vi "LV to ITX Retrieve_SE mode.vi"(0 "File or Folder Path":path=path "G:/My Drive/ansom/Data/MNK/SA03018F.20180502/4 - sweep B, Vsg IV superlattice", 5 "offset":i32, 7 "length":i32=1, 9 "index":T3={"A"=7, "B"=5, "C"=3, "D"=5, "E"=3, "N1"=2, "N2"=2, "N3"=3, "N4"=4, "A 1"=4, "A 2"=6, "C 1"=3, "C 2"=1, "E 2"=4}, 11 "stop":bool, 12 "File Type":T1) -> (1 "Spherical coordinates":dbl[][](array[numeric]), 2 "long":cluster{i32[], dbl[]}(graph), 3 "G vs T":cluster{dbl[], dbl[]}(graph), 4 "A vs B":cluster{dbl[], dbl[]}[](graph), 6 "C vs D":cluster{dbl[], dbl[]}[](graph), 8 "E( = A)":dbl[][](graph), 10 "N":cluster{"N1":dbl, "N2":dbl, "N3":dbl, "N4":dbl}={"N1"=17.9999, "N2"=17.9999, "N3"=0.00140599360448446, "N4"=0.001168874519263091} {"N4" format="%#_6p"; "N3" format="%#_6p"; "N2" format="%#_6p"; "N1" format="%#_6p"}, 13 "Index, Wavenames":string[][](table)=[["0", "'time.SA03018F.20180502.000000'\n"], ["1", "'temp.SA03018F.20180502.000000'\n"], ["2", "'B.SA03018F.20180502.000000'\n"], ["3", "'Vsource.SA03018F.20180502.000000'\n"], ["4", "'Lockin0.SA03018F.20180502.000000'\n"], ["5", "'Lockin1.SA03018F.20180502.000000'\n"], ["6", "'Lockin2.SA03018F.20180502.000000'\n"], ["7", "'Lockin3.SA03018F.20180502.000000'\n"], ["8", "'Lockin4.SA03018F.20180502.000000'\n"], ["9", "'Lockin5.SA03018F.20180502.000000'\n"], ["10", "'B_rate.SA03018F.20180502.000000'\n"], ["11", "'DC0.SA03018F.20180502.000000'\n"], ["12", "'DC1.SA03018F.20180502.000000'\n"], ["13", "'DC2.SA03018F.20180502.000000'\n"], ["14", "'DC3.SA03018F.20180502.000000'\n"], ["15", "'DC4.SA03018F.20180502.000000'\n"], ["16", "'DC5.SA03018F.20180502.000000'\n"], ["17", "'DC6.SA03018F.20180502.000000'\n"], ["18", "'DC7.SA03018F.20180502.000000'\n"], ["", ""]], 14 "Comments":string="IGOR\nX// Date: 5/3/2018 12:09 PM\nX// B=18T to -18T 0.5T steps\nX// T=30mK\nX// sweep Vsg -10mV --> 60mV, 0.25mV step\nX// Vsg=1.1V\nX// \nX// lockin settings:\nX// time constant =100ms\nX// order=2\nX// Fs=2000\nX// #s=5000\nX// \nX// superlattice\nX// \nX// lockin:\nX// 0: 4, voltage V+\nX// 1: 5, current 8mV AC 270uV DC, 0.4 Hz\nX// 2: 7, voltage V-\nX// 3: 3, current, drain\nX// 4: 2,\nX// 5: 1, \nX// appliedField= 18.000000\nX// appliedVsg= -0.010000\nX// B= 17.999900\n\n\n\n\n\n\n\n\n\n\n\n\n\n\n\n\n\n\n\n\n\n\n\n\n\n\n\n\n\n\n\n\n\n\n\n\n\n\n\n\nX \nX Display/R 'time.SA03018F.20180502.000000'\nX AppendToGraph 'temp.SA03018F.20180502.000000'\nX AppendToGraph 'B.SA03018F.20180502.000000'\nX AppendToGraph 'Vsource.SA03018F.20180502.000000'\nX AppendToGraph 'Lockin0.SA03018F.20180502.000000'\nX AppendToGraph 'Lockin1.SA03018F.20180502.000000'\nX AppendToGraph 'Lockin2.SA03018F.20180502.000000'\nX AppendToGraph 'Lockin3.SA03018F.20180502.000000'\nX AppendToGraph 'Lockin4.SA03018F.20180502.000000'\nX AppendToGraph 'Lockin5.SA03018F.20180502.000000'\nX AppendToGraph 'B_rate.SA03018F.20180502.000000'\nX AppendToGraph 'DC0.SA03018F.20180502.000000'\nX AppendToGraph 'DC1.SA03018F.20180502.000000'\nX AppendToGraph 'DC2.SA03018F.20180502.000000'\nX AppendToGraph 'DC3.SA03018F.20180502.000000'\nX AppendToGraph 'DC4.SA03018F.20180502.000000'\nX AppendToGraph 'DC5.SA03018F.20180502.000000'\nX AppendToGraph 'DC6.SA03018F.20180502.000000'\nX AppendToGraph 'DC7.SA03018F.20180502.000000'\nX Label bottom \"x label\"\nX Label left \"y label\"\nX ModifyGraph rgb('time.SA03018F.20180502.000000')=(65280,0,0)\nX ModifyGraph rgb('temp.SA03018F.20180502.000000')=(65280,18432,0)\nX ModifyGraph rgb('B.SA03018F.20180502.000000')=(65280,36864,0)\nX ModifyGraph rgb('Vsource.SA03018F.20180502.000000')=(65280,55296,0)\nX ModifyGraph rgb('Lockin0.SA03018F.20180502.000000')=(57344,65280,0)\nX ModifyGraph rgb('Lockin1.SA03018F.20180502.000000')=(37376,65280,0)\nX ModifyGraph rgb('Lockin2.SA03018F.20180502.000000')=(18944,65280,0)\nX ModifyGraph rgb('Lockin3.SA03018F.20180502.000000')=(512,65280,0)\nX ModifyGraph rgb('Lockin4.SA03018F.20180502.000000')=(0,65280,17920)\nX ModifyGraph rgb('Lockin5.SA03018F.20180502.000000')=(0,65280,36352)\nX ModifyGraph rgb('B_rate.SA03018F.20180502.000000')=(0,65280,54784)\nX ModifyGraph rgb('DC0.SA03018F.20180502.000000')=(0,57856,65280)\nX ModifyGraph rgb('DC1.SA03018F.20180502.000000')=(0,39424,65280)\nX ModifyGraph rgb('DC2.SA03018F.20180502.000000')=(0,20992,65280)\nX ModifyGraph rgb('DC3.SA03018F.20180502.000000')=(0,2560,65280)\nX ModifyGraph rgb('DC4.SA03018F.20180502.000000')=(17408,0,65280)\nX ModifyGraph rgb('DC5.SA03018F.20180502.000000')=(35840,0,65280)\nX ModifyGraph rgb('DC6.SA03018F.20180502.000000')=(54272,0,65280)\nX ModifyGraph rgb('DC7.SA03018F.20180502.000000')=(65280,0,58368)\nX Legend/C/N=text0/J \"\\\\s('time.SA03018F.20180502.000000') time\\r\\\\s('temp.SA03018F.20180502.000000') temp\\r\\\\s('B.SA03018F.20180502.000000') B\\r\\\\s('Vsource.SA03018F.20180502.000000') Vsource\\r\\\\s('Lockin0.SA03018F.20180502.000000') Lockin0\\r\\\\s('Lockin1.SA03018F.20180502.000000') Lockin1\\r\\\\s('Lockin2.SA03018F.20180502.000000') Lockin2\\r\\\\s('Lockin3.SA03018F.20180502.000000') Lockin3\\r\\\\s('Lockin4.SA03018F.20180502.000000') Lockin4\\r\\\\s('Lockin5.SA03018F.20180502.000000') Lockin5\\r\\\\s('B_rate.SA03018F.20180502.000000') B_rate\\r\\\\s('DC0.SA03018F.20180502.000000') DC0\\r\\\\s('DC1.SA03018F.20180502.000000') DC1\\r\\\\s('DC2.SA03018F.20180502.000000') DC2\\r\\\\s('DC3.SA03018F.20180502.000000') DC3\\r\\\\s('DC4.SA03018F.20180502.000000') DC4\\r\\\\s('DC5.SA03018F.20180502.000000') DC5\\r\\\\s('DC6.SA03018F.20180502.000000') DC6\\r\\\\s('DC7.SA03018F.20180502.000000') DC7\"\nX ModifyGraph mirror(bottom)=1\nX ModifyGraph width=216\nX ModifyGraph height={Aspect,0.6}\nX ModifyGraph Log(bottom)=0\nX ModifyGraph Log(left)=0\nX \n", 15 "E index vs Field":cluster{i32[], dbl[]}(graph))   [LabVIEW 2016, in "Retrieve and Visualize.lvclass"]
uses:
  Retrieve and Visualize.lvclass
  <vilib>/Utility/miscctls.llb/LVOffsetAndMultiplierTypeDef.ctl
  <userlib>/LevyLab/LV to ITX/Data/Typedefs/File Type--enum.ctl
  <vilib>/Analysis/3filter.llb/Savitzky-Golay Filter (DBL).vi
  <userlib>/LevyLab/XY Utilities/subVIs/Subset (single).vi
  <userlib>/LevyLab/XY Utilities/subVIs/Derivative (single).vi
  <userlib>/LevyLab/XY Utilities/subVIs/Decimate (single).vi
  <userlib>/LevyLab/Graph Utilities/graph_utilities.lvclass
  <vilib>/Analysis/NI_AALPro.lvlib
  <vilib>/Analysis/NI_AALBase.lvlib
  <userlib>/LevyLab/LV to ITX/Data/Data.lvclass
  <userlib>/LevyLab/XY Utilities/xy_utilities.lvlib
panel:
  out "Date":dbl format="%<%I:%M:%S %p\n%x>T"
  in  "Type":enum16{"dy/dx vs x", "dx/dy vs y"}(ring)
  in  "VRM mode":bool
  in  "Ring":u16(ring) items=["default", "DIFF"]
  in  "decimating factor":i32=1
  in  "decimate files":i32=1
  in  "side points":i32=6
  in  "fit points":dbl=10.0
  in  "Portion of data":cluster{dbl, dbl}(slide)={0.75, 0.25} scale=0.0..1.0
  in  "length 2":i32=2500
  in  "index 2":i32=1072
  out "Ns":T2(array[cluster])
  in  "SE?":bool=TRUE
  in  "D  is time?":bool
  in  "B is time?":bool
  in  "Ez name":string="Conductance (S)"
  in  "Ey name":string="BY (T)"
  in  "Ex name":string="Vsg (mV)"
  in  "C y name":string="voltage"
  in  "D x name":string="Vsg"
  in  "A y name":string="current"
  in  "B x name":string="Vsg"
  in  "recolor traces?":bool
  in  "Ex":T4={"Offset"=0.0, "Multiplier"=1.0}
  in  "Ey":T4={"Offset"=0.0, "Multiplier"=1.0}
  out "Path":path=path "G:/My Drive/ansom/Data/MNK/SA03018F.20180502/4 - sweep B, Vsg IV superlattice/SA03018F.20180502.000000.itx"
  out "counter":i32
  # "A1-A2\nC1-C2\nE-E2"
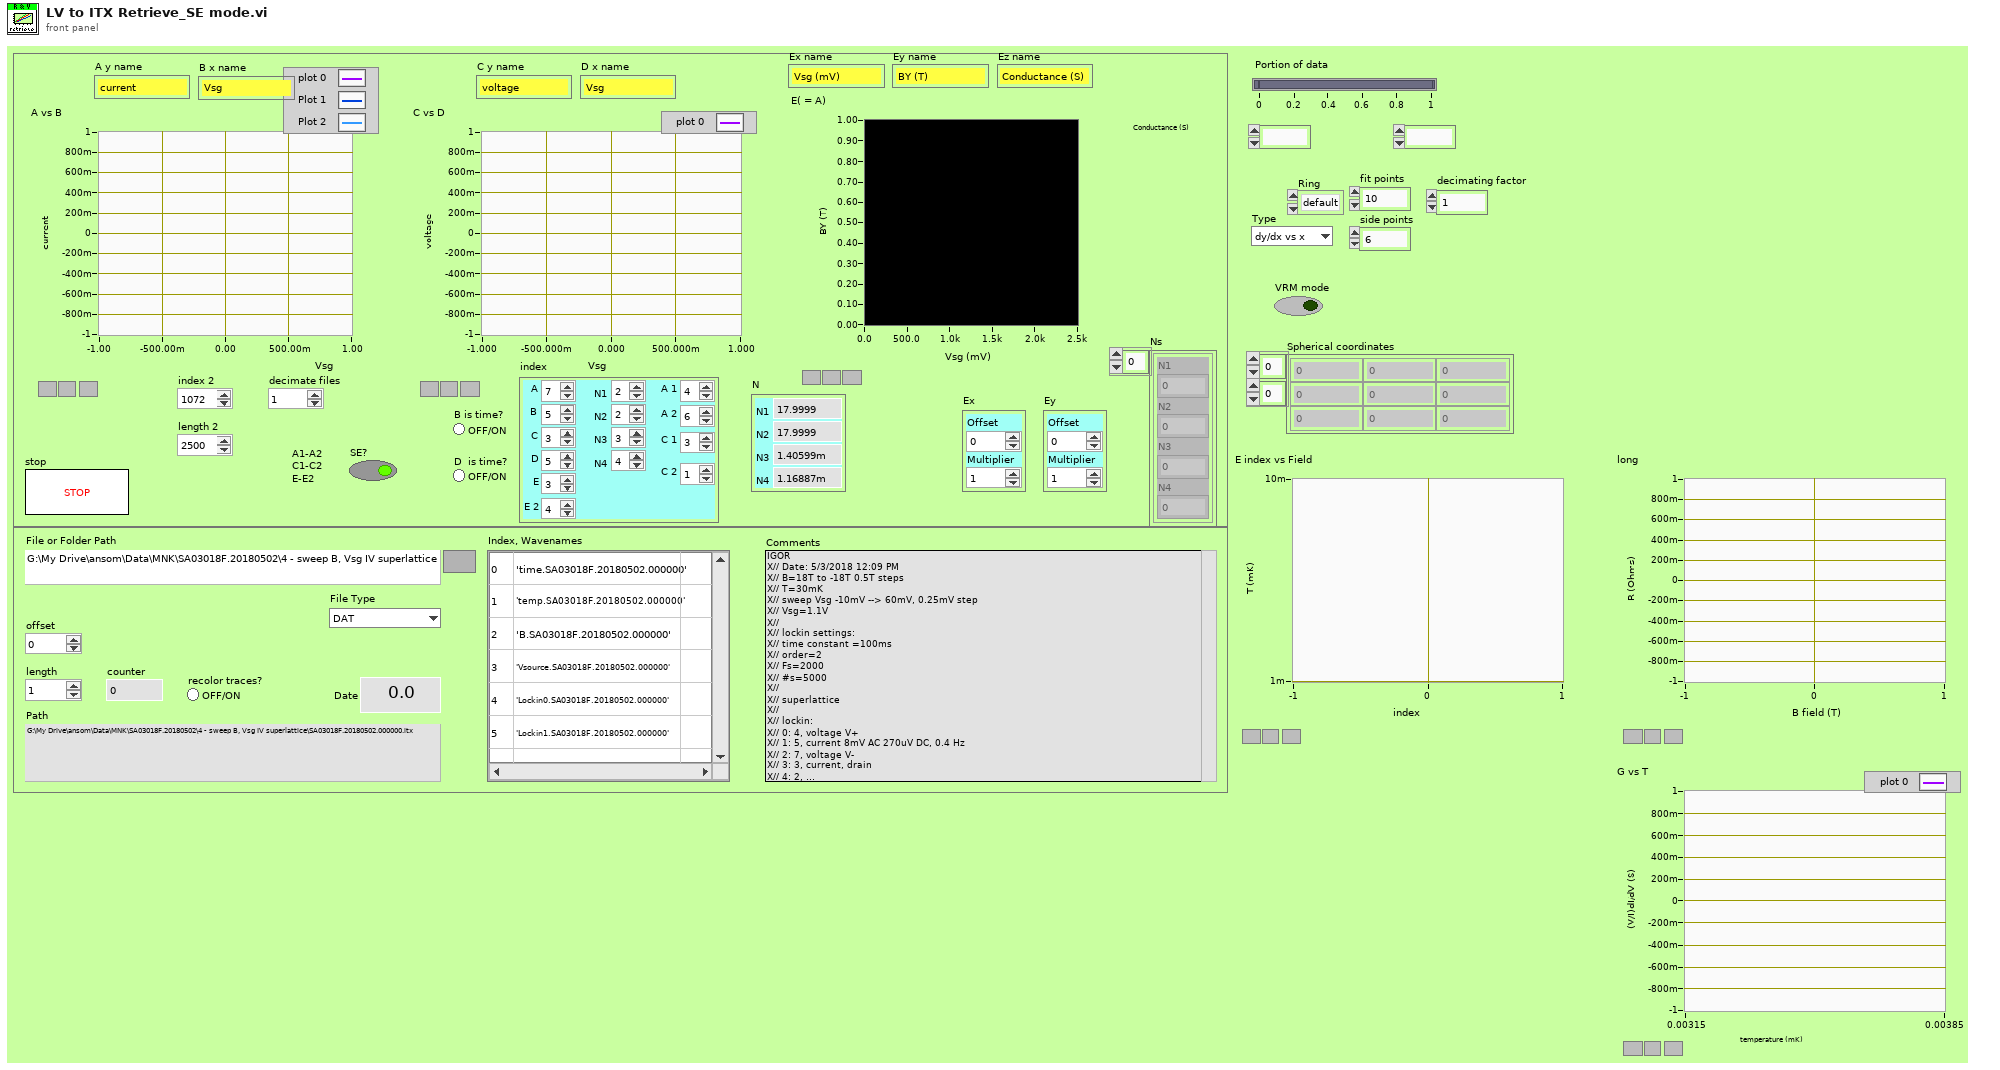
[diagram p1: front panel]
types:
  T1 = typedef "Data.lvclass/File Type--enum.ctl" = enum16{"DAT", "ITX", "TDMS", "VI"}
  T2 = cluster{"N1":dbl, "N2":dbl, "N3":dbl, "N4":dbl}[]
  T3 = cluster{"A":i32, "B":i32, "C":i32, "D":i32, "E":i32, "N1":i32, "N2":i32, "N3":i32, "N4":i32, "A 1":i32, "A 2":i32, "C 1":i32, "C 2":i32, "E 2":i32}
  T4 = typedef "LVOffsetAndMultiplierTypeDef.ctl" = cluster{"Offset":dbl, "Multiplier":dbl}
  T5 = typedef "Data.lvclass/Dictionary--cluster.ctl" = cluster{"key":string, "value":variant}
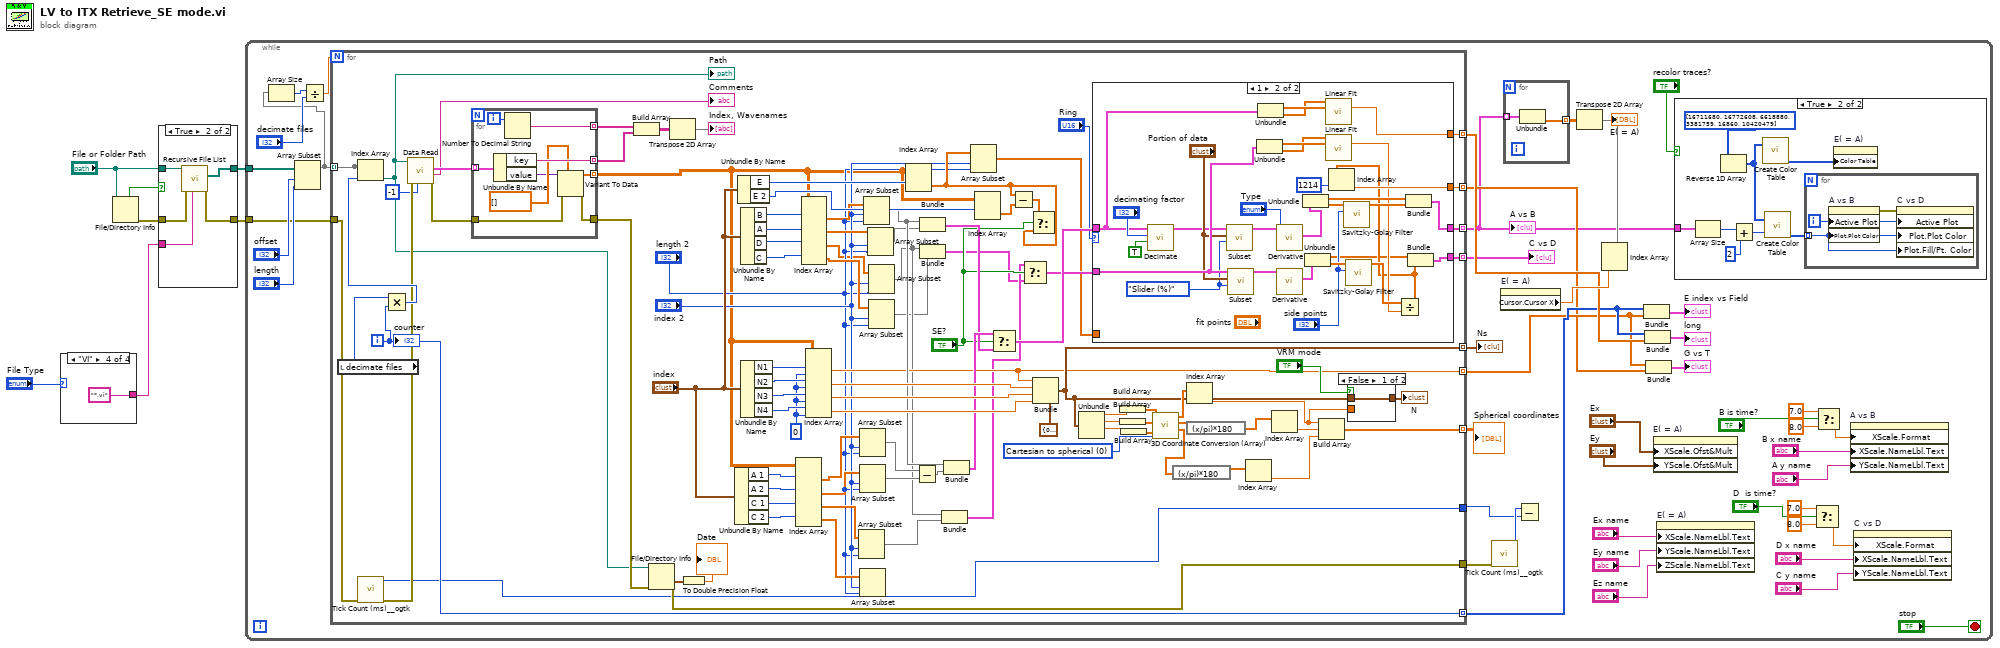
[diagram p0: block diagram]
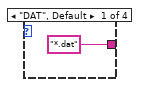
[diagram p2: hidden frame]
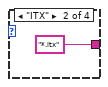
[diagram p3: hidden frame]
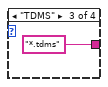
[diagram p4: hidden frame]
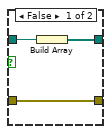
[diagram p5: hidden frame]
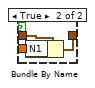
[diagram p7: hidden frame]
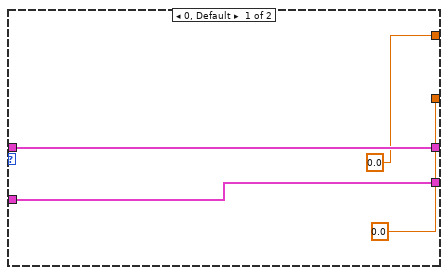
[diagram p8: hidden frame]
diagram:
  n1 = case shown="\"VI\"" "File Type" {
    tunnel: ["*.dat" ("pattern") "*.itx" ("pattern") "*.tdms" ("pattern") "*.vi" ("pattern")] -> w1
    frame "DAT", Default {
    }
    frame "ITX" {
    }
    frame "TDMS" {
    }
    frame "VI" {
    }
  }
  n2 = File/Directory Info(path="File or Folder Path") -> (directory=w5:bool, error out=w3:errorcluster)  [unwired: 1 in, 5 out]
  n3 = case shown="True" w5 {
    tunnel: [w14 w15] -> w6
    tunnel: "File or Folder Path" -> [w13 w19]
    tunnel: [w12 w18] -> w4
    tunnel: w3 -> [w12 w17]
    tunnel: w1 -> [_ w16]
    frame False {
      n4 = Build Array(w13) -> (w14:path[])
    }
    frame True {
      n5 = call <vilib>:"Recursive File List.vi"("pattern"=w16, "error in (no error)"=w17, "Folder Path"=w19) -> ("error out"=w18:errorcluster, "All Files in Dir"=w15:path[])  [unwired: 4 in, 3 out]
    }
  }
  n6 = while {
    tunnel: w6 -> [w41]
    tunnel: w4 -> [w24]
    stop <- "stop" stop-if-true
    n7 = Array Subset(array=w41, index="offset", length="length") -> (w37:path[])
    n8 = Array Size(array=w37) -> (size(s)=w40:i32)
    n9 = Divide(x=w40, y="decimate files") -> (x/y=w38:dbl)
    n10 = for {
      N: w38 -> [_]
      tunnel: w37 -> [w171]
      tunnel: [w171] -> _ mode=indexing
      tunnel: [w117] -> w25 mode=indexing
      tunnel: [w116] -> w26 mode=indexing
      tunnel: [w106] -> w44 mode=indexing
      tunnel: [w115] -> w42 mode=indexing
      tunnel: [w110] -> w34 mode=indexing
      tunnel: [w109] -> w27 mode=indexing
      tunnel: [w103] -> w31 mode=indexing
      tunnel: [w102] -> w30 mode=indexing
      tunnel: w24 -> [w84]
      tunnel: [w82] -> w22
      tunnel: [w81] -> w20
      i -> [w103]
      w132 = u16 0 items=["Cartesian to spherical", "spherical to Cartesian", "Cartesian to cylindrical", "cylindrical to Cartesian", "spherical to cylindrical", "cylindrical to spherical"] ("conversion type")
      w154 = 0 ("disabled index (col)")
      n11 = local read "decimate files"() -> (w113:i32)
      n12 = call <userlib>:"Tick Count (ms)__ogtk.vi"("error in (no error)"=w84) -> ("error out"=w83:errorcluster, "millisecond timer value"=w81:u32)  [unwired: 9 in]
      n13 = Multiply(x=w113, y=w103) -> (x*y=w114:i32)
      n14 = Index Array(array=w171, index=w114) -> (element=w79:path)
      "Path" <- w79
      n15 = call <userlib>:"Data Read.vi"("Append Index"=-1, "error in (no error)"=w83, "path"=w79) -> ("error out"=w89:errorcluster, "Notes"=→"Comments":string, "Data (Dictionary)"=w91:T5[])  [unwired: 5 in, 1 out]
      n16 = for {
        tunnel: [w179] -> w87 mode=indexing
        tunnel: w91 -> [w178] mode=indexing
        tunnel: [w177] -> w86 mode=indexing
        tunnel: [w175] -> w88 mode=indexing
        tunnel: w89 -> [w173]
        tunnel: [w172] -> w85
        i -> [w180]
        n17 = Unbundle By Name(w178) -> ("key"=w177:string, "value"=w174:variant)
        n18 = Number To Decimal String(number=w180) -> (decimal integer string=w179:string)  [unwired: 1 in]
        n19 = Variant To Data(error in=w173, type=dbl[] [], Variant=w174) -> (data=w175:dbl[], error out=w172:errorcluster)
      }
      n20 = Build Array(w87, w86) -> (w169:string[][])
      n21 = File/Directory Info(path=w79, error in=w85) -> (last mod=w78:timestamp, error out=w82:errorcluster)  [unwired: 5 out]
      n22 = Transpose 2D Array(2D array=w169) -> (transposed array=→"Index, Wavenames":string[][])
      n23 = To Double Precision Float(number=w78) -> (double precision float=→"Date":dbl)
      n24 = Unbundle By Name("index") -> ("A 1"=w153:i32, "A 2"=w152:i32, "C 1"=w151:i32, "C 2"=w150:i32)
      n25 = Unbundle By Name("index") -> ("E"=w162:i32, "E 2"=w145:i32)
      n26 = Unbundle By Name("index") -> ("B"=w161:i32, "A"=w160:i32, "D"=w159:i32, "C"=w158:i32)
      n27 = Unbundle By Name("index") -> ("N1"=w163:i32, "N2"=w164:i32, "N3"=w165:i32, "N4"=w166:i32)
      n28 = Index Array(array=w88, index (row) #1=w153, index (row) #2=w152, index (row) #3=w151, index (row) #4=w150) -> (element #1=w137:dbl[], element #2=w135:dbl[], element #3=w134:dbl[], element #4=w133:dbl[])  [unwired: 4 in]
      n29 = Index Array(array=w88, index (row) #1=w161, index (row) #2=w160, index (row) #3=w159, index (row) #4=w158) -> (element #1=w142:dbl[], element #2=w140:dbl[], element #3=w93:dbl[], element #4=w138:dbl[])  [unwired: 4 in]
      n30 = Index Array(array=w88, index (row) #1=w163, index (col) #1=w154, index (row) #2=w164, index (col) #2=w154, index (row) #3=w165, index (col) #3=w154, index (row) #4=w166, index (col) #4=w154) -> (element #1=w102:dbl, element #2=w156:dbl, element #3=w157:dbl, element #4=w168:dbl)
      n31 = Array Subset(array=w134, index="index 2", length="length 2") -> (w101:dbl[])
      n32 = Array Subset(array=w137, index="index 2", length="length 2") -> (w136:dbl[])
      n33 = Array Subset(array=w135, index="index 2", length="length 2") -> (w108:dbl[])
      n34 = Array Subset(array=w133, index="index 2", length="length 2") -> ()  [unwired: 1 out]
      n35 = Array Subset(array=w142, index="index 2", length="length 2") -> (w141:dbl[])
      n36 = Array Subset(array=w140, index="index 2", length="length 2") -> (w139:dbl[])
      n37 = Array Subset(array=w138, index="index 2", length="length 2") -> (w92:dbl[])
      n38 = Array Subset(array=w93, index="index 2", length="length 2") -> (w94:dbl[])
      n39 = Index Array(array=w88, index (row)=w162) -> (element=w98:dbl[])  [unwired: 1 in]
      n40 = Subtract(x=w136, y=w108) -> (x-y=w149:dbl[])
      n41 = Bundle(w141, w139) -> (w147:cluster{dbl[], dbl[]})  [unwired: 1 in]
      n42 = Bundle(w94, w92) -> (w99:cluster{dbl[], dbl[]})  [unwired: 1 in]
      n43 = Bundle(w94, w101) -> (w100:cluster{dbl[], dbl[]})  [unwired: 1 in]
      n44 = Bundle(w141, w149) -> (w148:cluster{dbl[], dbl[]})  [unwired: 1 in]
      n45 = Array Subset(array=w98, index="index 2", length="length 2") -> (w95:dbl[])
      n46 = Index Array(array=w88, index (row)=w145) -> (element=w144:dbl[])  [unwired: 1 in]
      n47 = Select(t=w148, s="SE?", f=w147) -> (s? t:f=w119:cluster{dbl[], dbl[]})
      n48 = Subtract(x=w98, y=w144) -> (x-y=w143:dbl[])
      n49 = Select(t=w100, s="SE?", f=w99) -> (s? t:f=w118:cluster{dbl[], dbl[]})
      n50 = Select(t=w143, s="SE?", f=w98) -> ()  [unwired: 1 out]
      n51 = Bundle(cluster=cluster{"N1":dbl, "N2":dbl, "N3":dbl, "N4":dbl} {"N1"=0.0, "N2"=0.0, "N3"=0.0, "N4"=0.0}, "N1"=w102, "N2"=w156, "N3"=w157, "N4"=w168) -> (w106:cluster{"N1":dbl, "N2":dbl, "N3":dbl, "N4":dbl})
      n52 = Unbundle(w106) -> ("N1"=w112:dbl, "N2"=w131:dbl, "N3"=w128:dbl)  [unwired: 1 out]
      n53 = case shown="1" "Ring" {
        tunnel: w119 -> [w188 w194]
        tunnel: w118 -> [w187 w200]
        tunnel: [w188 w203] -> w117
        tunnel: [w187 w202] -> w116
        tunnel: [0.0 w211] -> w110
        tunnel: [0.0 w208] -> w109
        tunnel: w95 -> [_ _]
        frame 0, Default {
        }
        frame 1 {
          w198 = enum16{"Slider (%)", "X[] min and max"}."Slider (%)" ("Subset Method")
          n54 = call-poly <userlib>:"Decimate.vi"("averaging (off)"=TRUE ("averaging"), "decimating factor (1)"="decimating factor", "XY-data"=w194) -> ("Decimated XY-data out"=w195:cluster{"X-array":dbl[], "Y-array":dbl[]})  [unwired: 7 in, 1 out]
          n55 = call-poly <userlib>:"Subset.vi"("Subset Method"=w198, "Subset Slider (%)"="Portion of data", "XY-data"=w195) -> ("XY-data out"=w192:cluster{"X-array":dbl[], "Y-array":dbl[]})  [unwired: 7 in, 1 out]
          n56 = call-poly <userlib>:"Subset.vi"("Subset Method"=w198, "Subset Slider (%)"="Portion of data", "XY-data"=w200) -> ("XY-data out"=w190:cluster{"X-array":dbl[], "Y-array":dbl[]})  [unwired: 7 in, 1 out]
          n57 = Unbundle(w200) -> (w212:dbl[], w207:dbl[])
          n58 = Unbundle(w194) -> (w213:dbl[], w210:dbl[])
          n59 = call-poly <userlib>:"Derivative.vi"("Type"="Type", "XY-data"=w192) -> ("Differential out"=w193:cluster{"X-array":dbl[], "Y-array":dbl[]})  [unwired: 7 in, 2 out]
          n60 = call-poly <userlib>:"Derivative.vi"("XY-data"=w190) -> ("Differential out"=w189:cluster{"X-array":dbl[], "Y-array":dbl[]})  [unwired: 8 in, 2 out]
          n61 = Unbundle(w193) -> ("X-array"=w218:dbl[], "Y-array"=w216:dbl[])
          n62 = Unbundle(w189) -> ("X-array"=w201:dbl[], "Y-array"=w215:dbl[])
          n63 = call <vilib>:"Linear Fit.vi"("Y"=w210, "X"=w213) -> ("slope"=w211:dbl)  [unwired: 9 in, 4 out]
          n64 = call <vilib>:"Linear Fit.vi"("Y"=w207, "X"=w212) -> ("slope"=w205:dbl)  [unwired: 9 in, 4 out]
          n65 = call-poly <vilib>:"Savitzky-Golay Filter.vi"("side points"="side points", "X"=w216) -> ("Filtered X"=w217:dbl[])  [unwired: 8 in, 1 out]
          n66 = call-poly <vilib>:"Savitzky-Golay Filter.vi"("side points"="side points", "X"=w215) -> ("Filtered X"=w206:dbl[])  [unwired: 8 in, 1 out]
          n67 = Divide(x=w206, y=w205) -> (x/y=w204:dbl[])
          n68 = Index Array(array=w204, index=1214) -> (element=w208:dbl)
          n69 = Bundle("X-array"=w218, "Filtered X"=w217) -> (w203:cluster{"X-array":dbl[], "Filtered X":dbl[]})  [unwired: 1 in]
          n70 = Bundle("X-array"=w201, w204) -> (w202:cluster{"X-array":dbl[], dbl[]})  [unwired: 1 in]
        }
      }
      n71 = Build Array(w112) -> (w130:dbl[])
      n72 = Build Array(w131) -> (w129:dbl[])
      n73 = Build Array(w128) -> (w127:dbl[])
      n74 = call <vilib>:"3D Coordinate Conversion (Array).vi"("conversion type"=w132, "Axis 3"=w127, "Axis 2"=w129, "Axis 1"=w130) -> ("Axis 3 Out"=w125:dbl[], "Axis 2 Out"=w126:dbl[], "Axis 1 Out"=w124:dbl[])  [unwired: 4 in, 1 out]
      n75 = expression code="(x/pi)*180" ("degrees to radians")(w125) -> (w122:dbl[])
      n76 = Index Array(array=w124) -> (element=w107:dbl)  [unwired: 1 in]
      n77 = expression code="(x/pi)*180" ("degrees to radians")(w126) -> (w123:dbl[])
      n78 = Index Array(array=w122) -> (element=w120:dbl)  [unwired: 1 in]
      n79 = Index Array(array=w123) -> (element=w121:dbl)  [unwired: 1 in]
      n80 = Build Array(w107, w121, w120) -> (w115:dbl[])
      n81 = case shown="False" "VRM mode" {
        tunnel: w107 -> [_ w184]
        tunnel: w106 -> [w181 w183]
        tunnel: [w181 w182] -> w105
        frame False {
        }
        frame True {
          n82 = Bundle By Name(cluster=w183, "N1"=w184) -> (w182:cluster{"N1":dbl, "N2":dbl, "N3":dbl, "N4":dbl})
        }
      }
      "N" <- w105
      "counter" <- w103
    }
    "Ns" <- w44
    "Spherical coordinates" <- w42
    "A vs B" <- w25
    "C vs D" <- w26
    n83 = call <userlib>:"Tick Count (ms)__ogtk.vi"("error in (no error)"=w22) -> ("millisecond timer value"=w21:u32)  [unwired: 9 in, 1 out]
    n84 = property on="E( = A)" class="IntGraph (strict)"() -> ("Cursor.Cursor X"=w35:dbl)  [unwired: 2 in, 2 out]
    n85 = for {
      tunnel: [w64] -> _ mode=indexing
      tunnel: [w65] -> w43 mode=indexing
      tunnel: w25 -> [w64] mode=indexing
      n86 = Unbundle(w64) -> ("Filtered X"=w65:dbl[])  [unwired: 1 out]
    }
    n87 = Subtract(x=w21, y=w20) -> ()  [unwired: 1 out]
    n88 = Transpose 2D Array(2D array=w43) -> (transposed array=w28:dbl[][])
    "E( = A)" <- w28
    n89 = Index Array(array=w28, index (row)=w35) -> ()  [unwired: 1 in, 1 out]
    n90 = Bundle(w31, w30) -> (→"E index vs Field":cluster{i32[], dbl[]})  [unwired: 1 in]
    n91 = Bundle(w31, w34) -> (→"long":cluster{i32[], dbl[]})  [unwired: 1 in]
    n92 = Bundle(w30, w27) -> (→"G vs T":cluster{dbl[], dbl[]})  [unwired: 1 in]
    n93 = property on="E( = A)" class="IntGraph (strict)"("XScale.Ofst&Mult"="Ex", "YScale.Ofst&Mult"="Ey") -> ()  [unwired: 2 in, 2 out]
    n94 = property on="E( = A)" class="IntGraph (strict)"("XScale.NameLbl.Text"="Ex name", "YScale.NameLbl.Text"="Ey name", "ZScale.NameLbl.Text"="Ez name") -> ()  [unwired: 2 in, 2 out]
    n95 = case shown="True" "recolor traces?" {
      tunnel: w25 -> [_ w68]
      frame False {
      }
      frame True {
        n96 = Array Size(array=w68) -> (size(s)=w69:i32)
        n97 = Reverse 1D Array(array=u32[] [16711680, 16772608, 6618880, 3381759, 16860, 10420479] ("color scale")) -> (reversed array=w67:u32[])
        n98 = Add(x=w69, y=2 ("x")) -> (x+y=w73:i32)
        n99 = call <userlib>:"Create Color Table.vi"("Colors []"=w67) -> ("Color Tbl"=w71:u32[])  [unwired: 1 in, 3 out]
        n100 = call <userlib>:"Create Color Table.vi"("Colors []"=w67, "Size (256)"=w73) -> ("Color Tbl"=w70:u32[])  [unwired: 3 out]
        n101 = for {
          tunnel: w70 -> [w74] mode=indexing
          i -> [w75]
          n102 = property on="A vs B" class="XYGraph (strict)"("Active Plot"=w75, "Plot.Plot Color"=w74) -> (error out=w76:errorcluster)  [unwired: 2 in, 1 out]
          n103 = property on="C vs D" class="XYGraph (strict)"(error in=w76, "Active Plot"=w75, "Plot.Plot Color"=w74, "Plot.Fill/Pt. Color"=w74) -> ()  [unwired: 1 in, 2 out]
        }
        n104 = property on="E( = A)" class="IntGraph (strict)"("Color Table"=w71) -> ()  [unwired: 2 in, 2 out]
      }
    }
    n105 = Select(t=7.0, s="D  is time?", f=8.0) -> (s? t:f=w49:dbl)
    n106 = Select(t=7.0, s="B is time?", f=8.0) -> (s? t:f=w50:dbl)
    n107 = property on="A vs B" class="XYGraph (strict)"("XScale.Format"=w50, "XScale.NameLbl.Text"="B x name", "YScale.NameLbl.Text"="A y name") -> ()  [unwired: 2 in, 2 out]
    n108 = property on="C vs D" class="XYGraph (strict)"("XScale.Format"=w49, "XScale.NameLbl.Text"="D x name", "YScale.NameLbl.Text"="C y name") -> ()  [unwired: 2 in, 2 out]
  }
